vi "Get Diagram Not Connected SubVI refs.vi"(11 "Diagram ref.":refnum<vi>) -> (3 "not connected SubVIs[]":refnum<vi>[](array[refnum]))   [LabVIEW 2014]
doc: "Returns Constant ownes by Diagram. So if you put numeric constants or string constants or now somewhere on diagram and they are not bounded any structure like WhileLoop or ForLoop, this function returns their references.\n\nFor now returns just DigitalNumericConstant and StringConstant refs as arrays."
panel:
  out "alltop objects refs[]":string[](array[string])
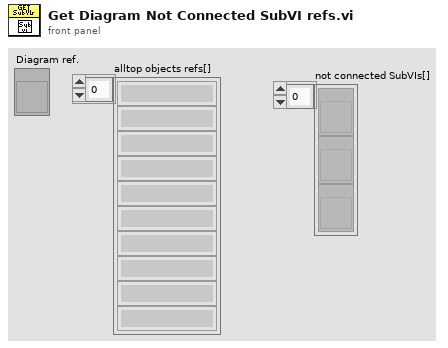
[diagram p1: front panel]
types:
  T1 = cluster{"terminals datatypes":string[][], "terminal\nconnected?":bool[], "terminal captions":string[], "term. count":i32, "terminal\nIsSource?":bool[], "SubVI name":string, "connected\nwires refs.":refnum<vi>[], "coerced dot?":bool[], "terminals[]":refnum<vi>[]}
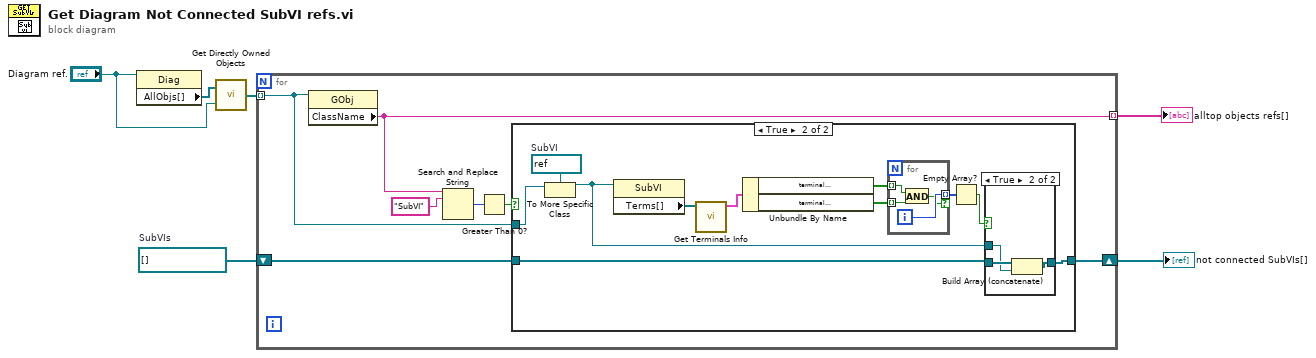
[diagram p0: block diagram]
diagram:
  w5 = refnum<vi>[] []  # SubVIs
  n1 = property on="Property Node" class="Diag"(reference="Diagram ref.") -> ("AllObjs[]"=w3:refnum<vi>[])  [unwired: 1 in, 2 out]
  n2 = call "Get Directly Owned Objects.vi"("Top Object"="Diagram ref.", "Nested Objects"=w3) -> ("Directly Owned Objects"=w1:refnum<vi>[])
  n3 = for {
    tunnel: w1 -> [w13] mode=indexing
    tunnel: [w11] -> w6 mode=indexing
    shift-right: [w7] -> w4
    shift-left: w5 -> [w12]
    n4 = property class="GObj"(reference=w13) -> ("ClassName"=w11:string)  [unwired: 1 in, 2 out]
    n5 = Search and Replace String(input string=w11, search string="SubVI") -> (number of replacements=w9:i32)  [unwired: 6 in, 3 out]
    n6 = Greater Than 0?(x=w9) -> (x > 0?=w8:bool)
    n7 = case shown="True" w8 {
      tunnel: w13 -> [_ w19]
      tunnel: [w14 w21] -> w7
      tunnel: w12 -> [w14 w25]
      frame False {
      }
      frame True {
        w24 = refnum<vi> refnum  # SubVI
        n8 = To More Specific Class(target class=w24, reference=w19) -> (specific class reference=w18:refnum<vi>)  [unwired: 1 in, 1 out]
        n9 = property class="SubVI"(reference=w18) -> ("Terms[]"=w23:refnum<vi>[])  [unwired: 1 in, 2 out]
        n10 = call "Get Terminals Info.vi"("Terms[]"=w23) -> ("output cluster"=w22:T1)  [unwired: 9 in, 1 out]
        n11 = Unbundle By Name(w22) -> ("terminal\nconnected?"=w17:bool[], "terminal\nIsSource?"=w16:bool[])
        n12 = for {
          tunnel: w17 -> [w28] mode=indexing
          tunnel: w16 -> [w29] mode=indexing
          tunnel: [w27] -> w15 mode=indexing if=w26
          i -> [w27]
          n13 = And(x=w28, y=w29) -> (x .and. y?=w26:bool)
        }
        n14 = Empty Array?(array=w15) -> (empty?=w20:bool)
        n15 = case shown="True" w20 {
          tunnel: w25 -> [w30 w32]
          tunnel: [w30 w33] -> w21
          tunnel: w18 -> [_ w31]
          frame False {
          }
          frame True {
            n16 = Build Array (concatenate)(w32, w31) -> (w33:refnum<vi>[])
          }
        }
      }
    }
  }
  "alltop objects refs[]" <- w6
  "not connected SubVIs[]" <- w4
